vi "Set Timer (End).vi"(7 "End Timer":T1 {"Start-Date (s)" format="%<%Y/%m/%d>T"; "Start-Time (s)" format="%<%H:%M>t"}, 8 "error in (no error)":errorcluster, 10 "Address (0)":i32, 11 "VISA resource name":refnum<visa-resource-name>) -> (0 "error out":errorcluster, 3 "VISA resource name out":refnum<visa-resource-name>)   [LabVIEW 2016, in "Environment Chamber.lvlib" / "Climatic Chamber.lvlib"]
doc: "<b>Timer writing</B>\n\nEdits the end timer."
uses:
  Climatic Chamber.lvlib
  Private/Type Defs/TimerNumber Enum.ctl
  Private/Type Defs/Start Mode Enum.ctl
  Private/Type Defs/Operation_Stop Mode Enum.ctl
  Private/Type Defs/Start_End Timer Cluster.ctl
panel:
  out "Error":bool
  out "NACK":bool
  out "ACK":bool
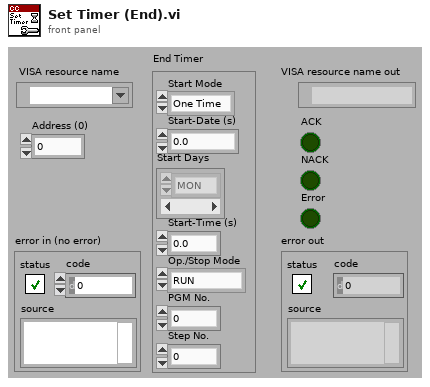
[diagram p1: front panel]
types:
  T1 = typedef "Environment Chamber.lvlib/Climatic Chamber.lvlib/Start_End Timer Cluster.ctl" = cluster{"Start Mode":T2, "Start-Date (s)":dbl, "Start Days":enum16{"MON", "TUE", "WED", "THU", "FRI", "SAT", "SUN"}[], "Start-Time (s)":dbl, "Op./Stop Mode":T3, "PGM No.":i32, "Step No.":i32}
  T2 = typedef "Environment Chamber.lvlib/Climatic Chamber.lvlib/Start Mode Enum.ctl" = enum16{"One Time", "Weekly", "Daily"}
  T3 = typedef "Environment Chamber.lvlib/Climatic Chamber.lvlib/Operation_Stop Mode Enum.ctl" = enum16{"RUN", "CONSTANT", "STANDBY", "OFF"}
  T4 = typedef "Environment Chamber.lvlib/Climatic Chamber.lvlib/TimerNumber Enum.ctl" = enum16{"Quick Timer", "Start Timer", "End Timer"}
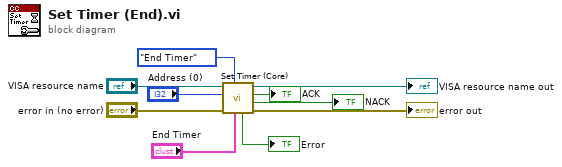
[diagram p0: block diagram]
diagram:
  n1 = call "Set Timer (Core).vi"("Start/End Timer"="End Timer", "Timer Number"=TimerNumber_Enum."End Timer", "error in (no error)"="error in (no error)", "Address (0)"="Address (0)", "VISA resource name"="VISA resource name") -> ("error out"=→"error out":errorcluster, "NACK"=→"NACK":bool, "ACK"=→"ACK":bool, "VISA resource name out"=→"VISA resource name out":refnum<visa-resource-name>, "Error"=→"Error":bool)  [unwired: 2 in]
